vi "SPI Slave Read Bytes From Buffer.vi"(7 "TimeOutMs":i32, 9 "pReadData":u8[](array[numeric])=array[4097 elements], 10 "SPIIndex":i32, 11 "DevHandle":i32) -> (1 "pReadData out":u8[](array[numeric]), 3 "function return":i32)   [LabVIEW 2010, in "usb2spi.lvlib"]
doc: "int WINAPI SPI_SlaveReadBytesFromBuffer(int DevHandle,int SPIIndex,unsigned char *pReadData,int TimeOutMs);"
uses:
  usb2spi.lvlib
  USB2XXX/trunk/USB2XXX/USB2XXX/vs2019/Release/USB2XXX.dll
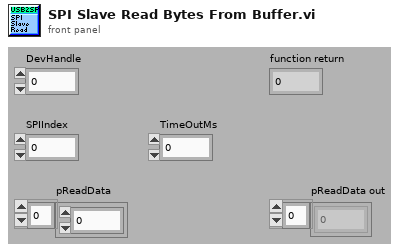
[diagram p1: front panel]
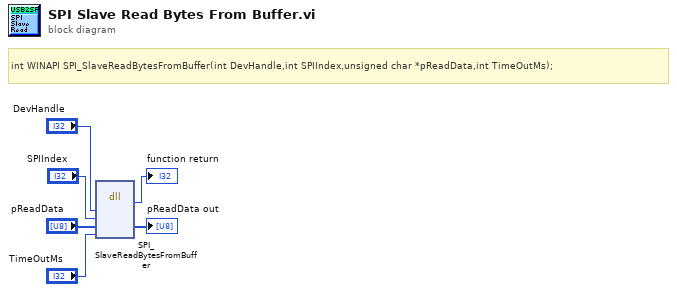
[diagram p0: block diagram]
diagram:
  # "int WINAPI SPI_SlaveReadBytesFromBuffer(int DevHandle,int SPIIndex,unsigned char *pReadData,int TimeOutMs);"
  n1 = dll-call lib="E:/Projects/USB2XXX/trunk/USB2XXX/USB2XXX/vs2019/Release/USB2XXX.*" fn="SPI_SlaveReadBytesFromBuffer"("DevHandle"="DevHandle", "SPIIndex"="SPIIndex", "pReadData"="pReadData", "TimeOutMs"="TimeOutMs") -> (→"function return":i32, "pReadData"=→"pReadData out":u8[])  [unwired: 6 in, 2 out]
